vi "getYear.vi"(8 "error in (no error)":errorcluster, 11 "WhichMonth in":refnum<class "WhichMonth.lvclass">) -> (0 "error out":errorcluster, 2 "YYYY":i32, 3 "WhichMonth out":refnum<class "WhichMonth.lvclass">)   [LabVIEW 2018, in "WhichMonth.lvclass"]
uses:
  WhichMonth.lvclass
  WhichMonth.lvclass/WhichMonth.ctl
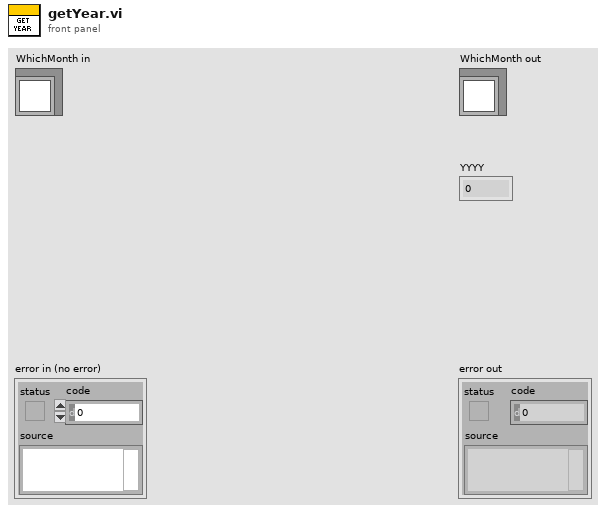
[diagram p1: front panel]
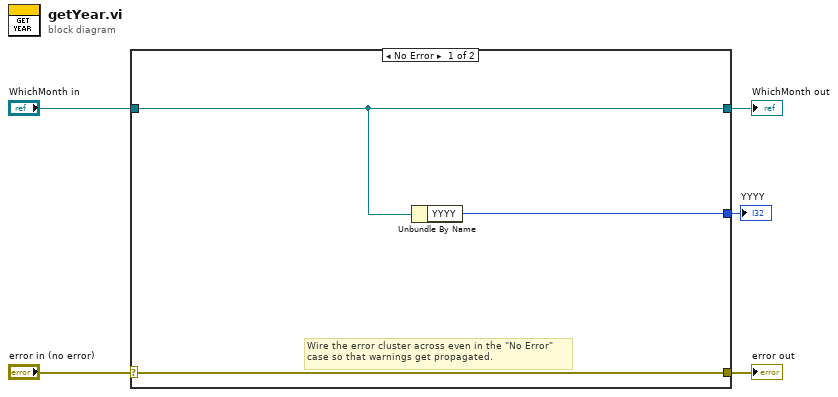
[diagram p0: block diagram]
diagram:
  n1 = case shown="No Error" "error in (no error)" {
    selector: "error in (no error)" -> [w8 w10]
    tunnel: [w8 w10] -> w4
    tunnel: [w7 w9] -> w2
    tunnel: "WhichMonth in" -> [w7 w9]
    tunnel: [w6 _] -> w1
    frame No Error {
      # "Wire the error cluster across even in the \"No Error\"\ncase so that warnings get propagated."
      n2 = Unbundle By Name(w7) -> ("YYYY"=w6:i32)
    }
    frame Error {
    }
  }
  "error out" <- w4
  "WhichMonth out" <- w2
  "YYYY" <- w1
